vi "getLVClassPrivateData.vi"(8 "error in":errorcluster, 11 "LVClass refnum":refnum<vi>) -> (0 "error out":errorcluster, 1 "Class Private Data Values":cluster{"Name":string, "Variant Data":variant}[](array[cluster]), 2 "Class Private Data VIRef":refnum<vi>, 3 "LVClass refnum out":refnum<vi>)   [LabVIEW 2017]
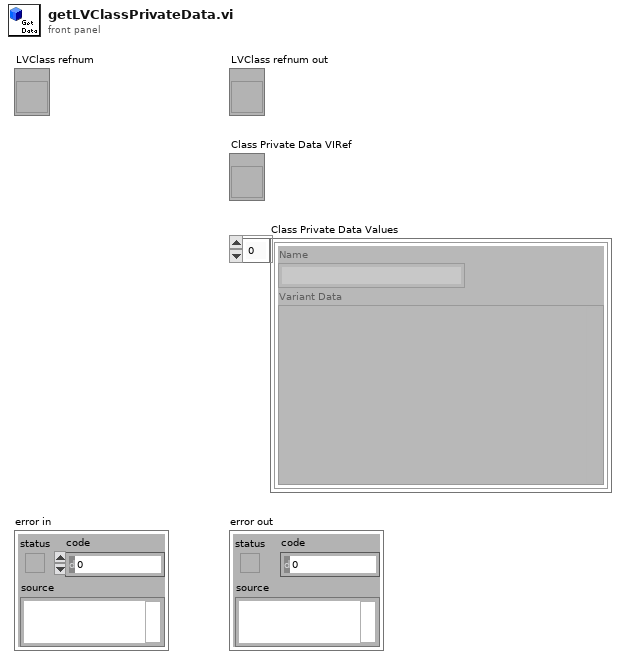
[diagram p1: front panel]
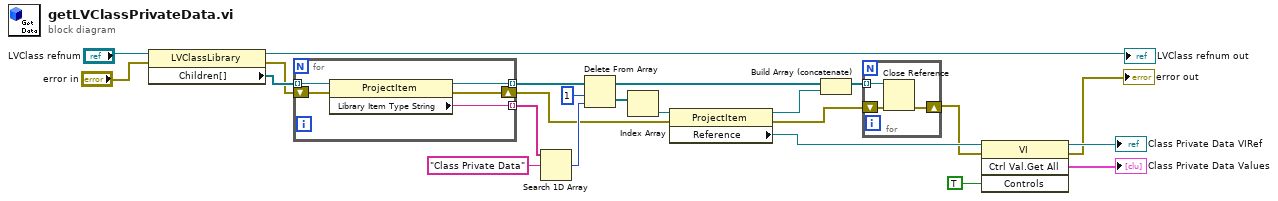
[diagram p0: block diagram]
diagram:
  n1 = property class="LVClassLibrary"(reference="LVClass refnum", error in="error in") -> (reference out=→"LVClass refnum out":refnum<vi>, error out=w8:errorcluster, "Children[]"=w23:refnum<vi>[])
  n2 = for {
    tunnel: w23 -> [w28] mode=indexing
    tunnel: [w27] -> w22 mode=indexing
    tunnel: [w26] -> w20 mode=indexing
    shift-right: [w24] -> w7
    shift-left: w8 -> [w25]
    n3 = property class="ProjectItem"(reference=w28, error in=w25) -> (reference out=w26:refnum<vi>, error out=w24:errorcluster, "Library Item Type String"=w27:string)
  }
  n4 = Search 1D Array(1D array=w22, element="Class Private Data" ("Library Item Type String")) -> (index of element=w18:i32)  [unwired: 1 out]
  n5 = Delete From Array(array=w20, length=1, index=w18) -> (deleted portion=w17:refnum<vi>[], array with subset deleted=w3:refnum<vi>[])
  n6 = Index Array(array=w17) -> (element=w16:refnum<vi>)  [unwired: 1 in]
  n7 = property class="ProjectItem"(reference=w16, error in=w7) -> (reference out=w4:refnum<vi>, error out=w1:errorcluster, "Reference"=w13:refnum<vi>)
  n8 = Build Array (concatenate)(w3, w4) -> (w2:refnum<vi>[])
  n9 = for {
    tunnel: w2 -> [w31] mode=indexing
    shift-right: [w29] -> w6
    shift-left: w1 -> [w30]
    n10 = Close Reference(reference=w31, error in (no error)=w30) -> (error out=w29:errorcluster)
  }
  n11 = invoke class="VI" method="Ctrl Val.Get All"(reference=w13, error in=w6, "Controls"=TRUE) -> (reference out=→"Class Private Data VIRef":refnum<vi>, error out=→"error out":errorcluster, "Get All Control Values Variant"=→"Class Private Data Values":cluster{"Name":string, "Variant Data":variant}[])  [unwired: 1 in, 1 out]
